vi "Setup Select Unwired Button.vi"(7 "Action":T2, 8 "error in (no error)":errorcluster, 9 "Display Items":T1[](array[typedef]), 10 "Properties for Tree In":T3(array[cluster]), 11 "Boolean in":refnum<vi>) -> (0 "error out":errorcluster)   [LabVIEW 2023]
uses:
  controls/action enum.ctl
  cluster/Cluster Element Description.ctl
panel:
  # "OR"
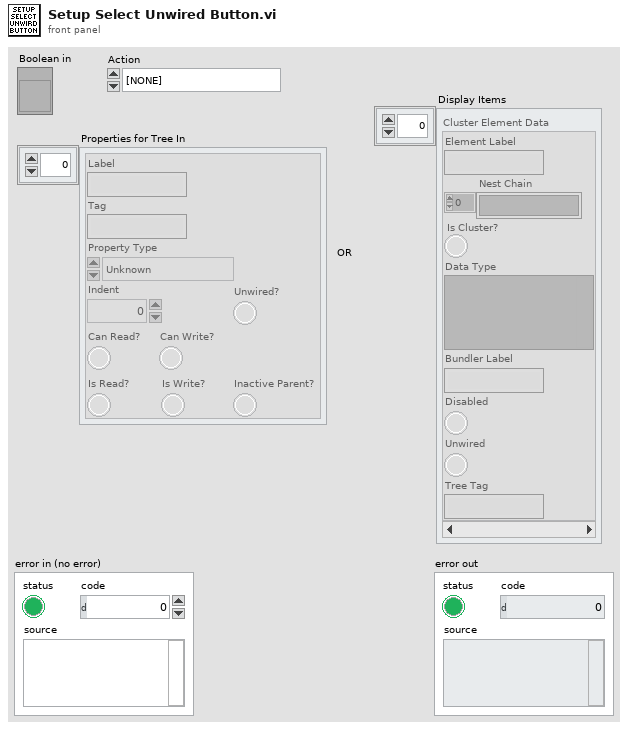
[diagram p1: front panel]
types:
  T1 = typedef "Cluster Element Description.ctl" = cluster{"Element Label":string, "Nest Chain":string[], "Is Cluster?":bool, "Data Type":variant, "Bundler Label":string, "Disabled":bool, "Unwired":bool, "Tree Tag":string}
  T2 = typedef "action enum.ctl" = enum16{"[NONE]", "Wire Bundle", "Wire Unbundle", "Terminal Unbundle", "Terminal Bundle", "Bundler Move Up", "Bundler Move Down", "Bundler Insert", "Bundler Remove", "Bundler Remove Unwired", "Bundler Rearrange", "In Place Insert", "In Place Remove", "In Place Remove Unwired", "In Place Rearrange", "Wire Properties", "Wire Method", "Terminal Properties", "Terminal Method", "Property Move Up", "Property Move Down", "Properties Insert", "Properties Remove", "Properties Remove Unwired", "Properties Rearrange", "Method Change", "Class For Constant", "Class For Control", "Class For Node", "Class Name to Clipboard"}
  T3 = cluster{"Label":string, "Tag":string, "Property Type":enum16{"Unknown", "Base", "Scripting", "Private", "Deprecated", "None", "Divider"}, "Indent":u16, "Can Read?":bool, "Can Write?":bool, "Is Read?":bool, "Is Write?":bool, "Inactive Parent?":bool, "Unwired?":bool}[]
  T4 = enum8{"Enabled", "Disabled", "Disabled and Grayed Out"}
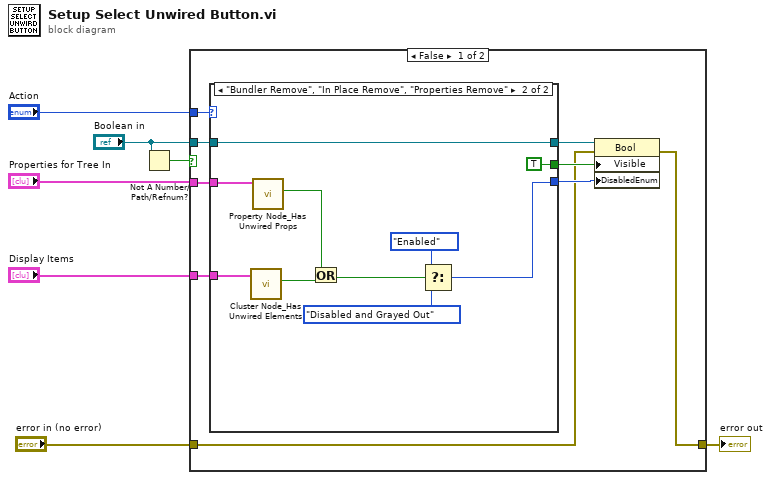
[diagram p0: block diagram]
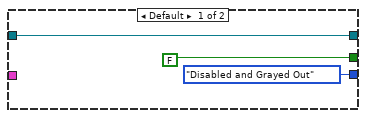
[diagram p2: hidden frame]
diagram:
  n1 = Not A Number/Path/Refnum?(number/path/refnum="Boolean in") -> (NaN/Path/Refnum?=w7:bool)
  n2 = case shown="False" w7 {
    tunnel: "Boolean in" -> [w15 _]
    tunnel: "Action" -> [w14 _]
    tunnel: "Properties for Tree In" -> [w12 _]
    tunnel: "Display Items" -> [w11 _]
    tunnel: "error in (no error)" -> [w9 w30]
    tunnel: [w8 w30] -> w1
    frame False {
      n3 = case shown="\"Bundler Remove\", \"In Place Remove\", \"Properties Remove\"" w14 {
        tunnel: [w18 w29] -> w16
        tunnel: w15 -> [w18 w29]
        tunnel: [FALSE TRUE] -> w13
        tunnel: w12 -> [_ w28]
        tunnel: w11 -> [_ w27]
        tunnel: [T4."Disabled and Grayed Out" ("Disabled") w21] -> w10
        frame Default {
        }
        frame "Bundler Remove", "In Place Remove", "Properties Remove" {
          n4 = call "Cluster Node_Has Unwired Elements.vi"("Display Items"=w27) -> ("Has unwired properties?"=w26:bool)  [unwired: 9 in, 1 out]
          n5 = call "Property Node_Has Unwired Props.vi"("Properties for Tree In"=w28) -> ("Has unwired properties?"=w25:bool)  [unwired: 9 in, 1 out]
          n6 = Or(x=w25, y=w26) -> (x .or. y?=w22:bool)
          n7 = Select(t=T4."Enabled" ("Disabled"), s=w22, f=T4."Disabled and Grayed Out" ("Disabled")) -> (s? t:f=w21:T4)
        }
      }
      n8 = property class="Bool"(reference=w16, error in=w9, "Visible"=w13, "DisabledEnum"=w10) -> (error out=w8:errorcluster)  [unwired: 1 out]
    }
    frame True {
    }
  }
  "error out" <- w1
